vi "Word_Update_Table.vi"(0 "Word.Tables":refnum<k7>, 1 "Word._Application":refnum<k7>, 5 "value":string[][](array[string]), 7 "table index":i16=-1, 9 "start":cluster{"row":i32, "column":i32}, 11 "error in":errorcluster) -> (15 "error out":errorcluster)   [LabVIEW 2017, in "NI_ReportGenerationToolkit.lvlib"]
uses:
  <vilib>/addons/_office/NI_ReportGenerationToolkit.lvlib
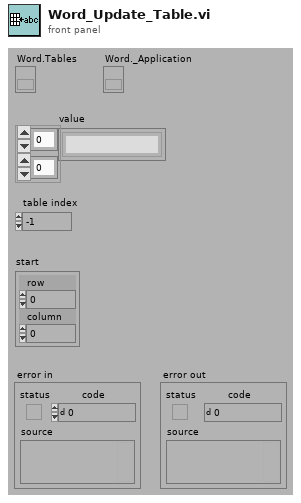
[diagram p1: front panel]
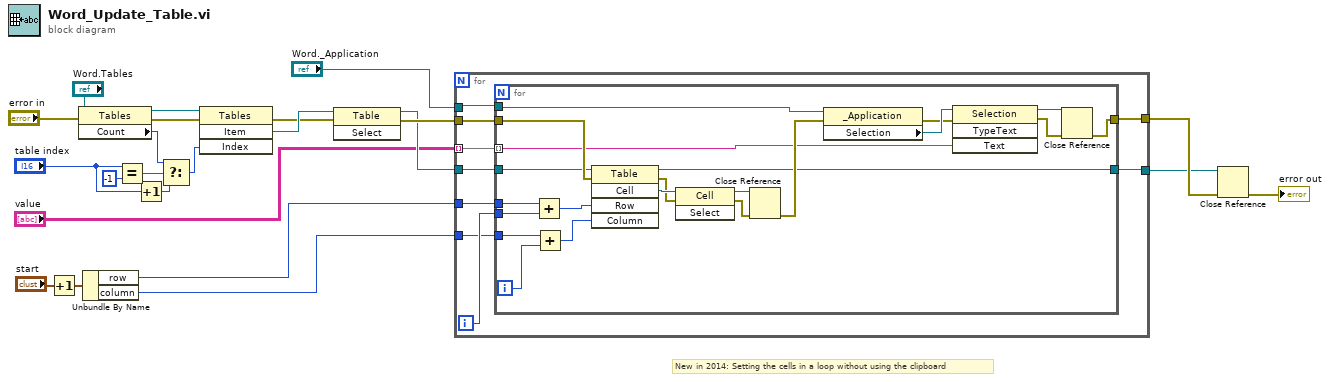
[diagram p0: block diagram]
diagram:
  # "New in 2014: Setting the cells in a loop without using the clipboard"
  n1 = Increment(x="start") -> (x+1=w12:cluster{"row":i32, "column":i32})
  n2 = property class="Tables"(reference="Word.Tables", error in="error in") -> (reference out=w17:refnum<k7>, error out=w15:errorcluster, "Count"=w19:i32)
  n3 = Unbundle By Name(w12) -> ("row"=w4:i32, "column"=w3:i32)
  n4 = Equal?(x="table index", y=i16 -1) -> (x = y?=w21:bool)
  n5 = Increment(x="table index") -> (x+1=w13:i16)
  n6 = Select(t=w19, s=w21, f=w13) -> (s? t:f=w14:i32)
  n7 = invoke class="Tables" method="Item"(reference=w17, error in=w15, "Index"=w14) -> (error out=w7:errorcluster, "Item"=w8:refnum<k7>)  [unwired: 1 in, 2 out]
  n8 = invoke class="Table" method="Select"(reference=w8, error in=w7) -> (reference out=w9:refnum<k7>, error out=w10:errorcluster)  [unwired: 1 in, 1 out]
  n9 = for {
    tunnel: "value" -> [w32] mode=indexing
    tunnel: [w31] -> w1
    tunnel: [w30] -> w2
    tunnel: w10 -> [w28]
    tunnel: "Word._Application" -> [w27]
    tunnel: w9 -> [w26]
    tunnel: w4 -> [w25]
    tunnel: w3 -> [w24]
    i -> [w29]
    n10 = for {
      tunnel: w32 -> [w44] mode=indexing
      tunnel: [w48] -> w31
      tunnel: [w41] -> w30
      tunnel: w29 -> [w38]
      tunnel: w28 -> [w47]
      tunnel: w27 -> [w46]
      tunnel: w26 -> [w45]
      tunnel: w25 -> [w36]
      tunnel: w24 -> [w35]
      i -> [w37]
      n11 = Add(x=w36, y=w38) -> (x+y=w34:i32)
      n12 = Add(x=w35, y=w37) -> (x+y=w33:i32)
      n13 = invoke class="Table" method="Cell"(reference=w45, error in=w47, "Row"=w34, "Column"=w33) -> (reference out=w48:refnum<k7>, error out=w52:errorcluster, "Cell"=w53:refnum<k7>)  [unwired: 1 in, 2 out]
      n14 = invoke class="Cell" method="Select"(reference=w53, error in=w52) -> (reference out=w49:refnum<k7>, error out=w51:errorcluster)  [unwired: 1 in, 1 out]
      n15 = Close Reference(reference=w49, error in (no error)=w51) -> (error out=w50:errorcluster)
      n16 = property class="_Application"(reference=w46, error in=w50) -> (error out=w39:errorcluster, "Selection"=w40:refnum<k7>)  [unwired: 1 out]
      n17 = invoke class="Selection" method="TypeText"(reference=w40, error in=w39, "Text"=w44) -> (reference out=w42:refnum<k7>, error out=w43:errorcluster)  [unwired: 1 in, 2 out]
      n18 = Close Reference(reference=w42, error in (no error)=w43) -> (error out=w41:errorcluster)
    }
  }
  n19 = Close Reference(reference=w1, error in (no error)=w2) -> (error out=→"error out":errorcluster)
